vi "Enable Load Extension.vi"(8 "error in (no error)":errorcluster, 10 "Enable":bool=TRUE, 11 "Connection in":refnum<class "Connection.lvclass">) -> (0 "error out":errorcluster, 3 "Connection out":refnum<class "Connection.lvclass">)   [LabVIEW 2023, in "SQLite.lvlib" / "Connection.lvclass"]
doc: "Sets the Busy Timeout of the Connection: the time opertions such as \"Step\" will wait when the database is locked by another connection before returning an error."
uses:
  Connection.lvclass
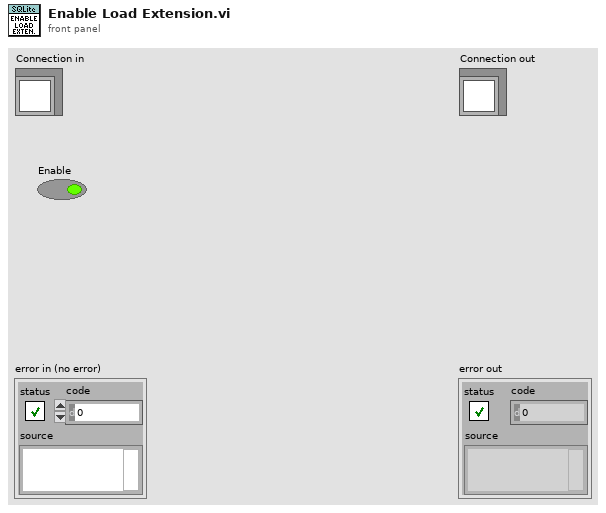
[diagram p1: front panel]
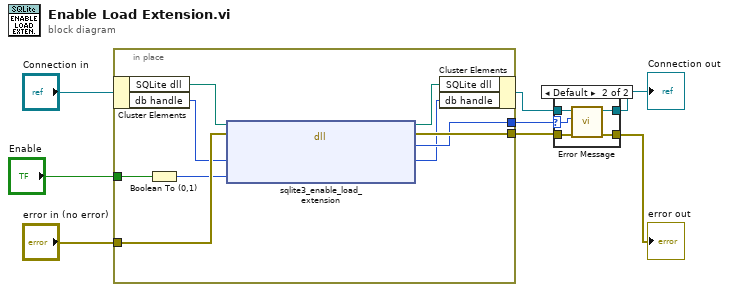
[diagram p0: block diagram]
diagram:
  n1 = in-place {
    in-place-border: "error in (no error)" -> [w17]
    in-place-border: "Enable" -> [w16]
    in-place-border: [w15] -> w6
    in-place-border: [w14] -> w5
    n2 = in-place-cluster #1("Connection in") -> ("SQLite dll"=w10:path, "db handle"=w13:u64)
    n3 = Boolean To (0,1)(Boolean=w16) -> (0, 1=w9:i16)
    n4 = dll-call lib="C:/LabVIEW_JDP/Support/SQLite/SQL Connection/sqlite3.dll" fn="sqlite3_enable_load_extension"(path in=w10, error in=w17, "db handle"=w13, "on(1)/off(0)"=w9) -> (path out=w11:path, error out=w15:errorcluster, "return code"=w14:i32, "db handle"=w12:u64)  [unwired: 2 in]
    n5 = in-place-cluster #1("SQLite dll"=w11, "db handle"=w12) -> (w2:refnum<class "Connection.lvclass">)
  }
  n6 = case shown="Default" w5 {
    selector: w5 -> [_ w21]
    tunnel: [w18 w24] -> w1
    tunnel: w6 -> [w19 w23]
    tunnel: [w19 w22] -> w4
    tunnel: w2 -> [w18 w20]
    frame 0 {
      # "No Error"
    }
    frame Default {
      n7 = call "Error Message.vi"("error in (no error)"=w23, "error code"=w21, "Connection in"=w20) -> ("error out"=w22:errorcluster, "Connection out"=w24:refnum<class "Connection.lvclass">)  [unwired: 7 in]
    }
  }
  "error out" <- w4
  "Connection out" <- w1
